vi "Autonomous Independent-old.vi"() -> ()   [LabVIEW 2013]
doc: "This VI is called when autonomous begins, and will automatically be terminated when autonomous ends. You can carry out timed or sensor driven robot movement independently without needing to return to the caller."
uses:
  <vilib>/Rock Robotics/WPI/Solenoid/WPI_SolenoidValue.ctl
  Robot Global Data.vi
  <vilib>/Rock Robotics/WPI/Solenoid/WPI_SolenoidSetEnum.vi
  <vilib>/Rock Robotics/WPI/RobotDrive/WPI_RobotDriveArcadeDrive_Standard(NoSaturation).vi
  <vilib>/Rock Robotics/WPI/RobotDrive/WPI_RobotDriveGetSetRefNum.vi
  <vilib>/Rock Robotics/WPI/Joystick/WPI_JoystickGetSetRefNum.vi
  <vilib>/addons/control/pid/NI_PID_pid.lvlib
  <vilib>/addons/control/pid/pid.llb/PID (DBL).vi
  TargetType.ctl
panel:
  out "Go now or wait?":enum16{"Go Now", "Wait"}(ring)
  out "Stop Time":u32=1000
  in  "stop":bool
  out "Drive Forward Time":u32=1000
  out "Shoot Time":u32=1000
  out "Right? (T)":bool
  out "Position":T1
  in  "Launcher State":enum16{"Shoot", "Out", "Retract"}(ring)
  in  "Shooter Extended Time":u32=500
  out "Shooter Tick":u32
  out "Check Target Time":u32=5000
  out "Left?":bool
  out "Raise Arms Time":u32=1500
  in  "Up Position":dbl format="%.2f"
  out "Close Arms Time":u32=250
  out "Lower Arms Time":u32=1500
  in  "Down Position":dbl format="%.2f"
  out "Open Arms Time":u32=250
  in  "Auton State":T2(ring)
  out "Tick at start of Auton":u32
  out "Current Movement, for debugging":T3 {"Y Joystick Value" scale=1.0..-1.0; "X Joystick Value" scale=-1.0..1.0}
  in  "Array of robot movements":T4(array[cluster]) {"Y Joystick Value" scale=1.0..-1.0; "X Joystick Value" scale=-1.0..1.0}
  # "Be sure to right-click and choose Data Operations>>Make Current Value default if you want to save the array values with the VI"
  # "Main State Machine"
  # "Shooter State Machine"
  # "Disabled"
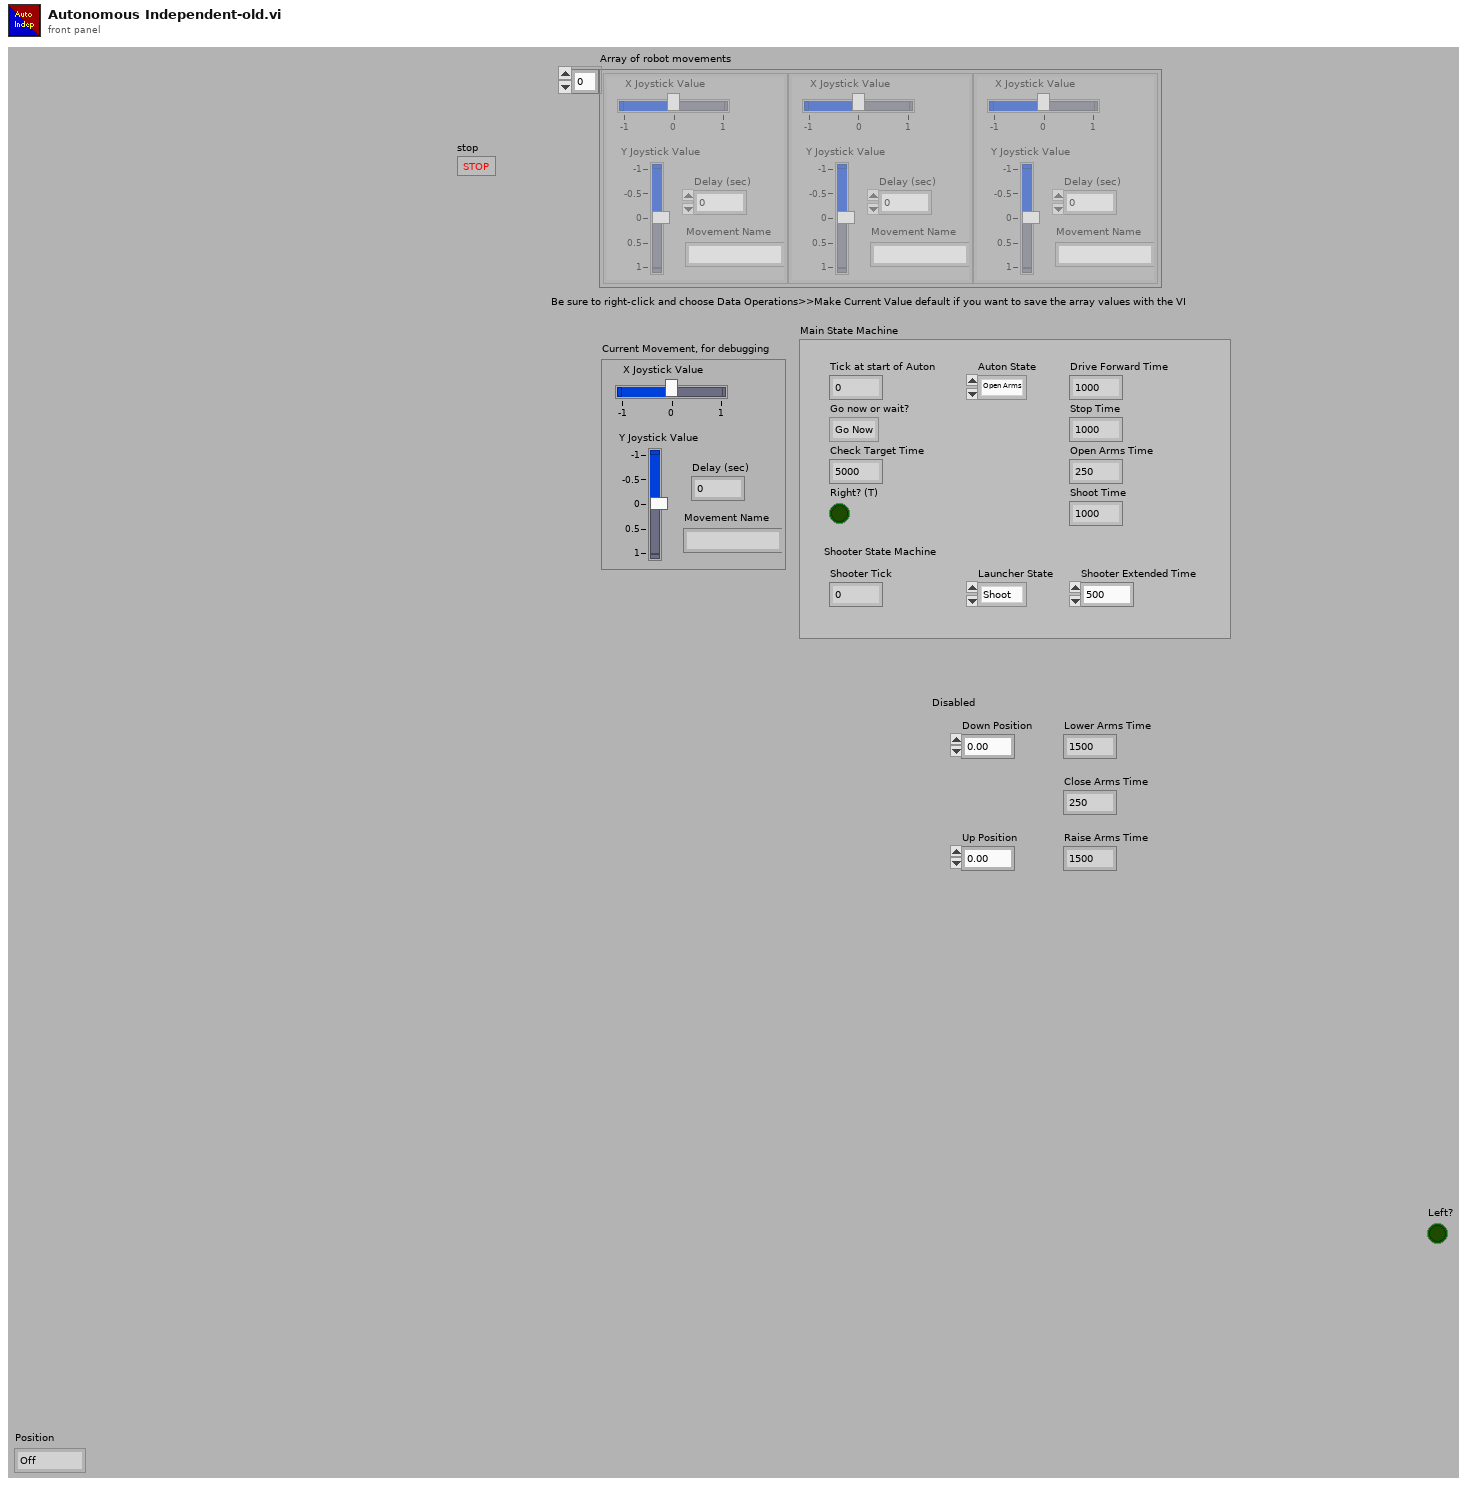
[diagram p1: front panel]
types:
  T1 = typedef "WPI_SolenoidValue.ctl" = enum16{"Off", "On", "Forward", "Reverse"}
  T2 = enum16{"Open Arms", "Lower Arms", "Close Arms", "Raise Arms", "Check Target", "Shoot", "Drive Forward", "Stop"}
  T3 = cluster{"X Joystick Value":dbl, "Y Joystick Value":dbl, "Delay (sec)":dbl, "Movement Name":string}
  T4 = cluster{"X Joystick Value":dbl, "Y Joystick Value":dbl, "Delay (sec)":dbl, "Movement Name":string}[]
  T5 = typedef "WPI_JoystickDevRef.ctl" = cluster{"Device":T6}
  T6 = typedef "WPI_JoystickDeviceEnum.ctl" = enum16{"USB 1", "USB 2", "USB 3", "USB 4", "Kinect 1", "Kinect 2"}
  T7 = cluster{"axis 1 (x)":dbl, "axis 2 (y)":dbl, "axis 3 (throttle)":dbl, "axis 4":dbl, "axis 5":dbl, "axis 6":dbl}
  T8 = typedef "TargetType.ctl" = enum16{"Not Hot", "Hot"}
  T9 = enum16{"Open Arms", "Lower Arms", "Close Arms", "Raise Arms", "Check Target", "Shoot", "Drive Forward"}
  T10 = cluster{"proportional gain (Kc)":dbl, "integral time (Ti, min)":dbl, "derivative time (Td, min)":dbl}
  T11 = typedef "WPI_SolenoidDevRef.ctl" = cluster{"DevStatus":errorcluster, "Solenoid Module":T12, "Forward Solenoid Channel":T13, "Reverse Solenoid Channel":T13}
  T12 = typedef "FPGA_TypedefSolenoidModule.ctl" = enum16{"Solenoid Module 1", "Solenoid Module 2"}
  T13 = typedef "WPI_SolenoidChannel.ctl" = enum8{"Solenoid 1", "Solenoid 2", "Solenoid 3", "Solenoid 4", "Solenoid 5", "Solenoid 6", "Solenoid 7", "Solenoid 8", "Invalid"}
  T14 = enum16{"Target Right", "No Target", "Target Left"}
  T15 = typedef "WPI_RobotDriveDevRef.ctl" = cluster{"DevStatus":errorcluster, "Motors[]":T16[], "Square Inputs":bool, "Max Output":dbl, "Isochronous":bool}
  T16 = typedef "WPI_MotorControlDeviceRef.ctl" = cluster{"DeviceStatus":errorcluster, "Type":enum16{"PWM", "CAN"}, "PWM":cluster{"Digital Module":T17, "PWM Channel":T18, "DeadBand":T19}, "CAN":cluster{"Device Number":u8, "Control Mode":T20, "Semaphore":T21, "Max Vout":dbl}, "Invert":bool, "TransformRef":T22, "InvTransformRef":T22}
  T17 = typedef "FPGA_TypedefDigitalModule.ctl" = enum16{"Digital Module 1", "Digital Module 2"}
  T18 = typedef "FPGA_DIOPWMChannel.ctl" = enum8{"PWM 1", "PWM 2", "PWM 3", "PWM 4", "PWM 5", "PWM 6", "PWM 7", "PWM 8", "PWM 9", "PWM 10", "Invalid"}
  T19 = typedef "WPI_PWMDeadband.ctl" = cluster{"Name":string, "maxPositivePwm":i32, "minPositivePwm":i32, "centerPwm":i32, "maxNegativePwm":i32, "minNegativePwm":i32, "angularRange":u16}
  T20 = typedef "WPI_CANJaguar_ControlMode.ctl" = enum8{"Percent VBus", "Current", "Speed", "Position", "Voltage"}
  T21 = typedef "Semaphore RefNum" = refnum<k1>
  T22 = typedef "WPI_PWMTransform_ConPane.ctl" = refnum<vi>
  T23 = cluster{"Distance (ft)":dbl, "Target Center (-1 to 1)":cluster{"X":dbl, "Y":dbl}, "Left":bool, "State":T8}
  T24 = typedef "WPI_AnalogChannelDevRef.ctl" = cluster{"DevStatus":errorcluster, "Analog Module":T25, "Analog Channel":T26}
  T25 = typedef "FPGA_TypedefAnalogModule.ctl" = enum16{"Analog Module 1", "Analog Module 2"}
  T26 = typedef "FPGA_AIChannel.ctl" = enum8{"AI 1", "AI 2", "AI 3", "AI 4", "AI 5", "AI 6", "AI 7", "AI 8", "Invalid"}
  T27 = typedef "WPI_DigitalInputDevRef.ctl" = cluster{"DevStatus":errorcluster, "DIO Channel":T28, "Digital Module":T17}
  T28 = typedef "FPGA_DIOChannel.ctl" = enum8{"DIO 1", "DIO 2", "DIO 3", "DIO 4", "DIO 5", "DIO 6", "DIO 7", "DIO 8", "DIO 9", "DIO 10", "DIO 11", "DIO 12", "DIO 13", "DIO 14", "Invalid"}
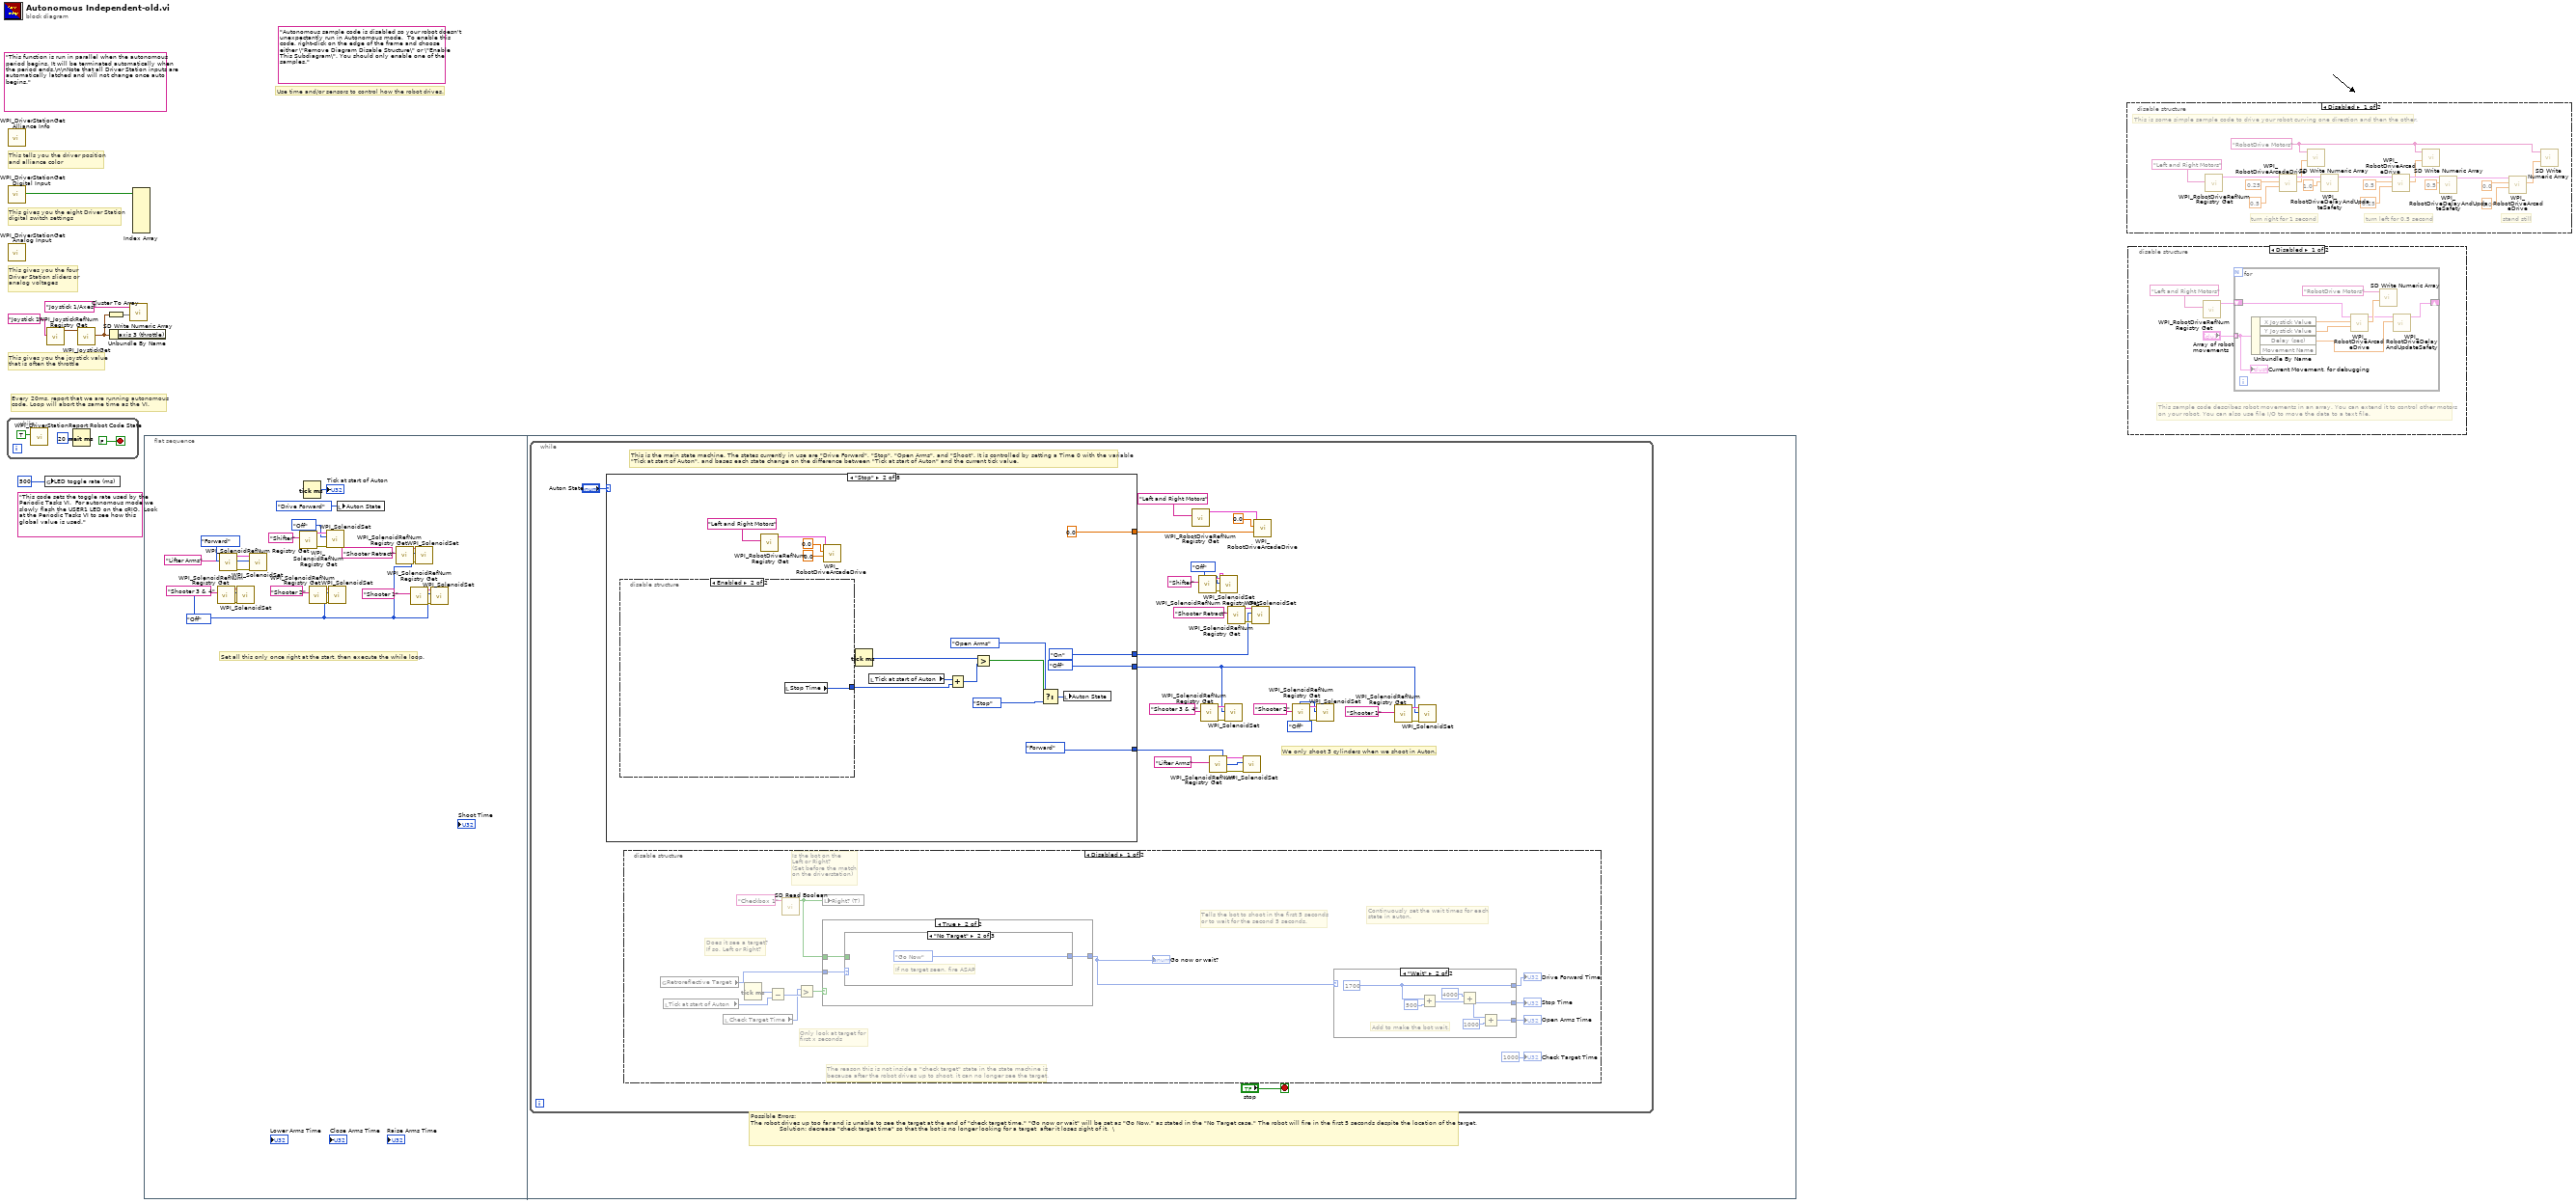
[diagram p0: block diagram]
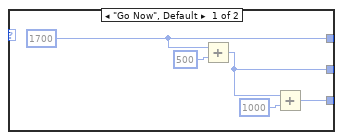
[diagram p2: hidden frame]
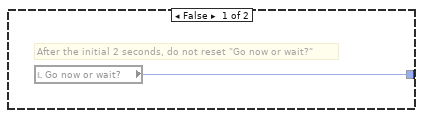
[diagram p3: hidden frame]
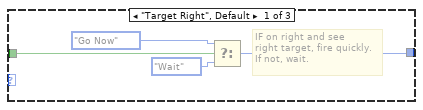
[diagram p4: hidden frame]
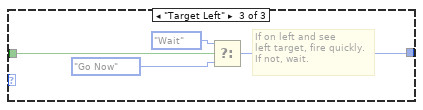
[diagram p5: hidden frame]
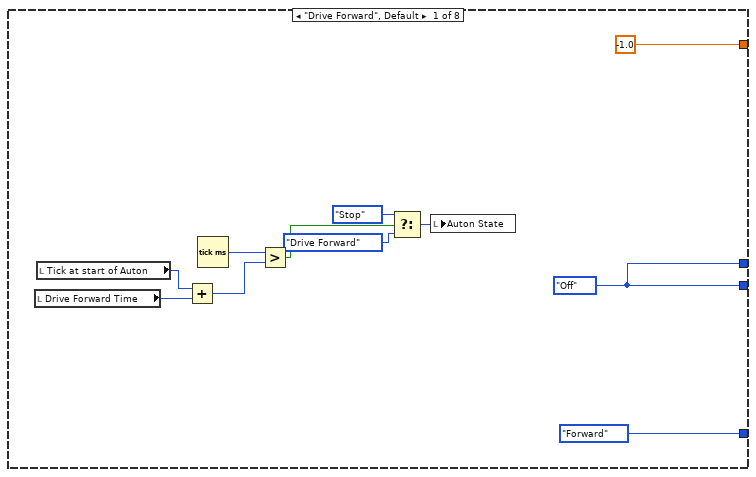
[diagram p7: hidden frame]
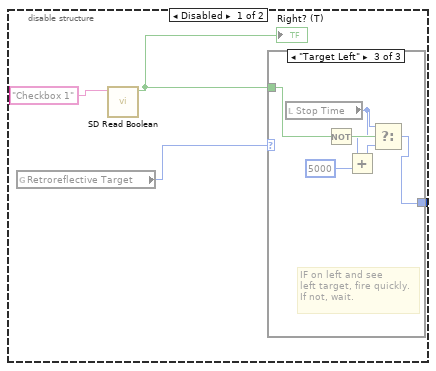
[diagram p8: hidden frame]
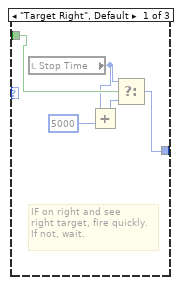
[diagram p9: hidden frame]
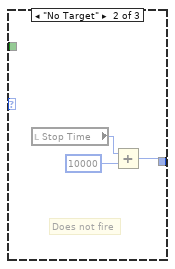
[diagram p10: hidden frame]
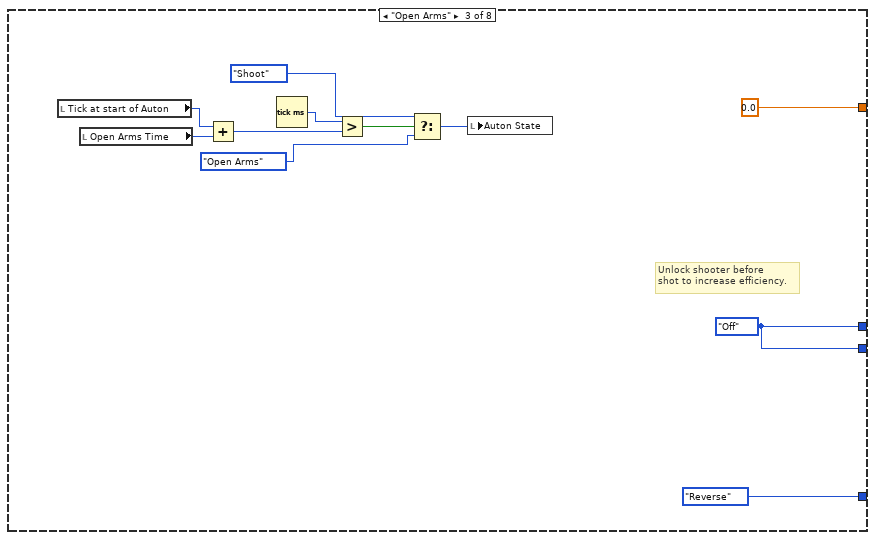
[diagram p11: hidden frame]
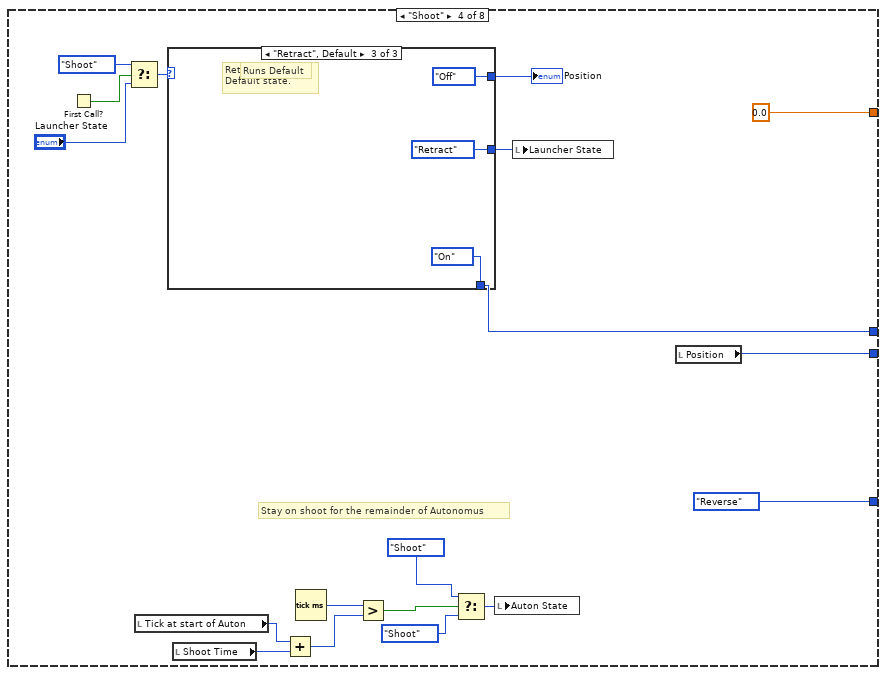
[diagram p12: hidden frame]
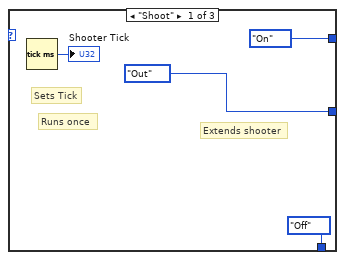
[diagram p13: hidden frame]
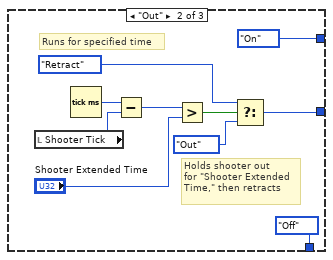
[diagram p14: hidden frame]
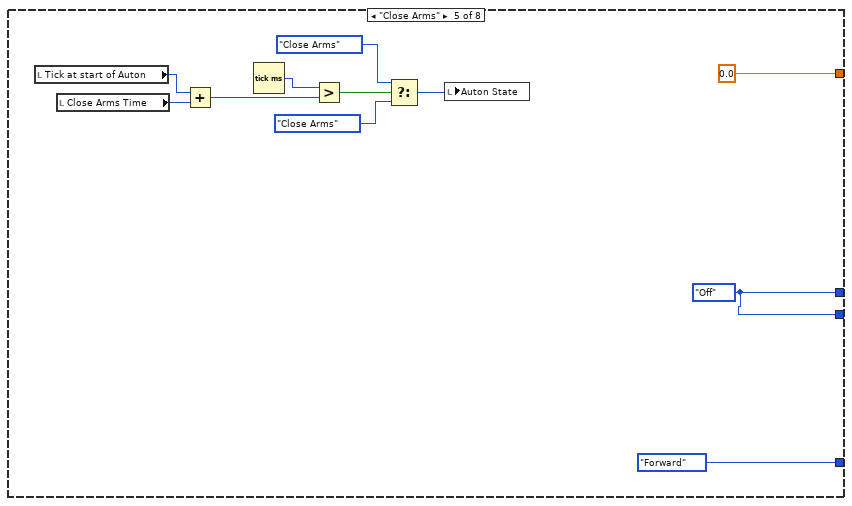
[diagram p15: hidden frame]
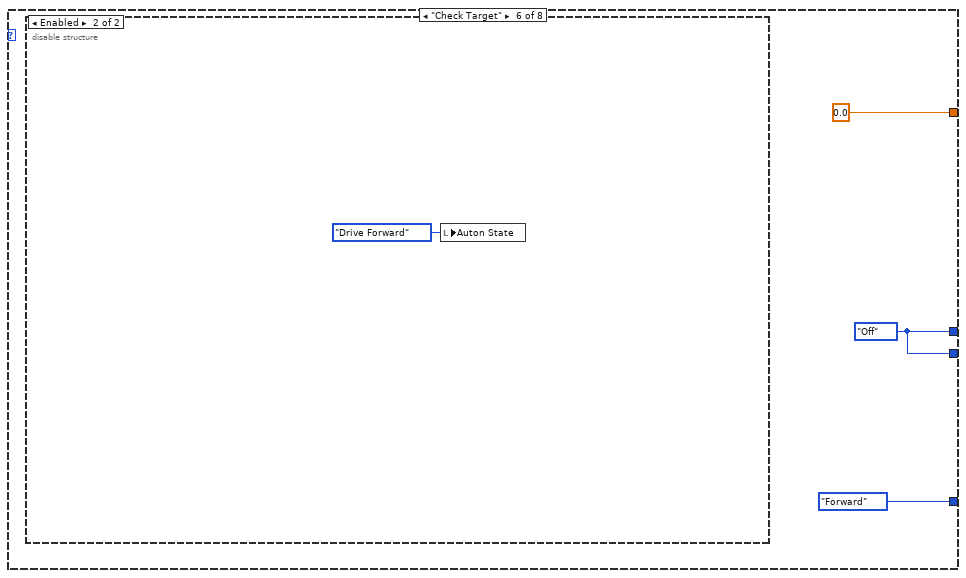
[diagram p16: hidden frame]
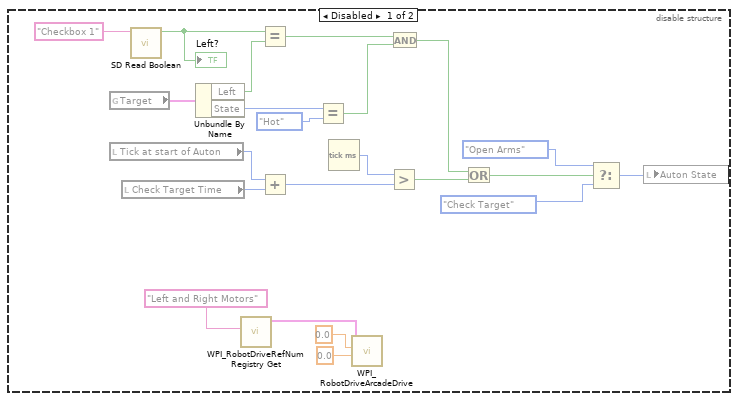
[diagram p17: hidden frame]
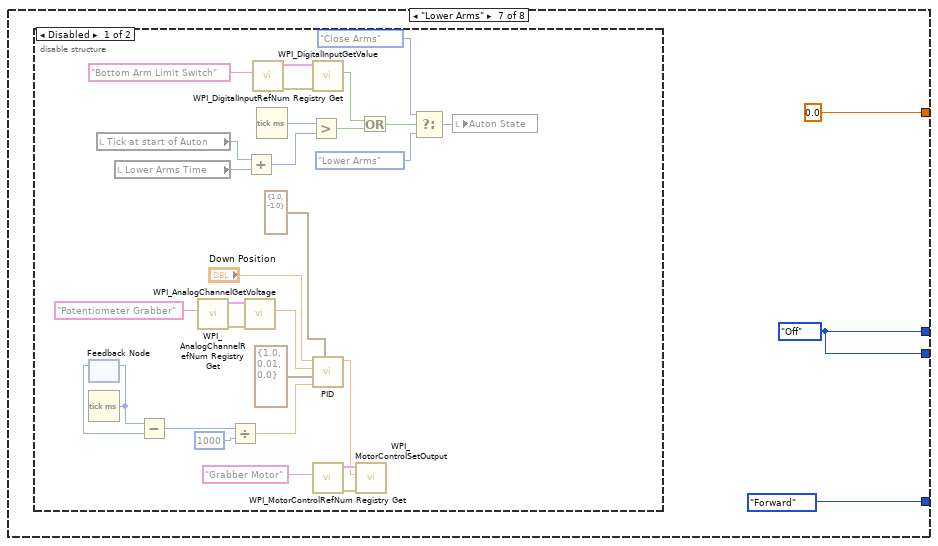
[diagram p18: hidden frame]
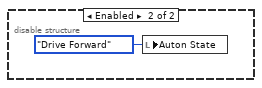
[diagram p19: hidden frame]
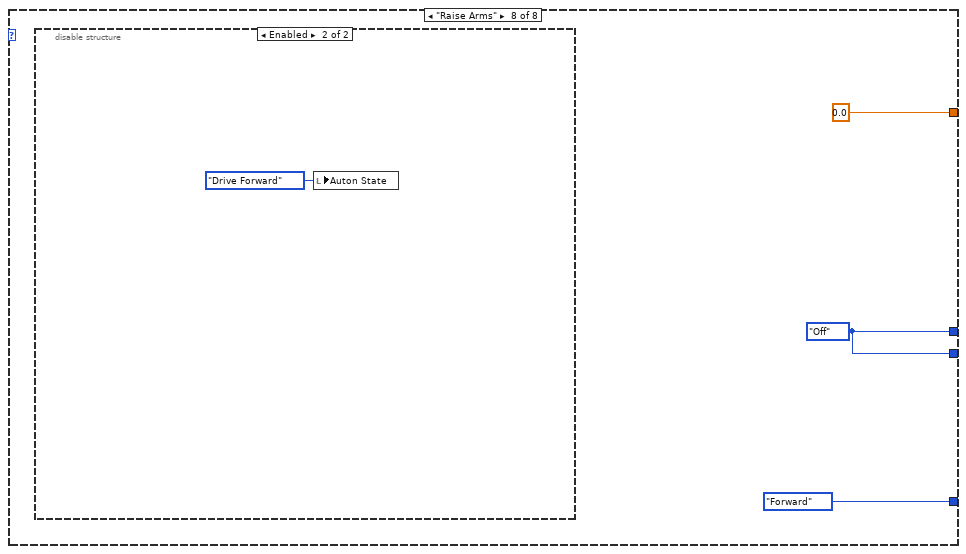
[diagram p20: hidden frame]
diagram:
  (unwired) "This code sets the toggle rate used by the Periodic Tasks VI.  For autonomous mode we slowly flash the USER1 LED on the cRIO.  Look at the Periodic Tasks VI to see how this global value is used."
  (unwired) "Autonomous sample code is disabled so your robot doesn't unexpectantly run in Autonomous mode.  To enable this code, right-click on the edge of the frame and choose either \"Remove Diagram Disable Structure\" or \"Enable This Subdiagram\". You should only enable one of the samples."
  (unwired) "This function is run in parallel when the autonomous period begins. It will be terminated automatically when the period ends.\n\nNote that all Driver Station inputs are automatically latched and will not change once auto begins."
  # "Every 20ms, report that we are running autonomous\ncode. Loop will abort the same time as the VI."
  # "This gives you the joystick value\nthat is often the throttle"
  # "Use time and/or sensors to control how the robot drives."
  # "This tells you the driver position\nand alliance color"
  # "This gives you the eight Driver Station\ndigital switch settings"
  # "This gives you the four\nDriver Station sliders or\nanalog voltages"
  n1 = while {
    stop <- FALSE stop-if-true
    n2 = call <vilib>:"WPI_DriverStationReport Robot Code State.vi"("Autonomous"=TRUE) -> ()  [unwired: 10 in, 1 out]
    n3 = Wait (ms)(milliseconds to wait=u32 20) -> ()  [unwired: 1 out]
  }
  n4 = call <vilib>:"WPI_DriverStationGet Alliance Info.vi"() -> ()  [unwired: 12 out]
  n5 = call <vilib>:"WPI_DriverStationGet Digital Input.vi"() -> ("Driver Station Digital Input (1-8)"=w7:bool[])  [unwired: 11 out]
  n6 = call <vilib>:"WPI_DriverStationGet Analog Input.vi"() -> ()  [unwired: 12 out]
  n7 = global write "Robot Global Data.vi" "LED toggle rate (ms)"(u32 500 ("LED ms toggle rate")) -> ()
  n8 = call <vilib>:"WPI_JoystickRefNum Registry Get.vi"("refnum name"="Joystick 1") -> ("JoystickDevRef"=w5:T5)  [unwired: 1 in, 9 out]
  n9 = call <vilib>:"WPI_JoystickGet.vi"("JoystickDevRef"=w5) -> ("Axes"=w2:T7)  [unwired: 1 in, 5 out]
  n10 = Cluster To Array(cluster=w2) -> (array=w3:dbl[])
  n11 = Unbundle By Name(w2) -> ()  [unwired: 1 out]
  n12 = call <vilib>:"SD Write Numeric Array.vi"("Numeric Array"=w3, "Name"="Joystick 1/Axes") -> ()  [unwired: 8 in, 2 out]
  n13 = Index Array(array=w7) -> ()  [unwired: 8 in, 8 out]
  n14 = flat-sequence {
    frame #0 {
      w19 = WPI_SolenoidValue."Off" ("x")
      # "Set all this only once right at the start, then execute the while loop."
      n15 = call <vilib>:"WPI_SolenoidRefNum Registry Get.vi"("refnum name"="Shooter 3 & 4") -> ("error out"=w26:errorcluster, "SolenoidDevRef"=w30:T11)  [unwired: 9 in]
      n16 = call <vilib>:"WPI_SolenoidRefNum Registry Get.vi"("refnum name"="Lifter Arms") -> ("error out"=w13:errorcluster, "SolenoidDevRef"=w14:T11)  [unwired: 9 in]
      n17 = call-poly <vilib>:"WPI_SolenoidSet.vi"("error in (no error)"=w26, "Value"=w19, "SolenoidDevRef"=w30) -> ()  [unwired: 7 in, 2 out]
      n18 = call-poly <vilib>:"WPI_SolenoidSet.vi"("error in (no error)"=w13, "Value"=WPI_SolenoidValue."Forward", "SolenoidDevRef"=w14) -> ()  [unwired: 7 in, 2 out]
      n19 = call <vilib>:"WPI_SolenoidRefNum Registry Get.vi"("refnum name"="Shifter") -> ("error out"=w17:errorcluster, "SolenoidDevRef"=w16:T11)  [unwired: 9 in]
      n20 = Tick Count (ms)() -> (millisecond timer value=→"Tick at start of Auton":u32)
      n21 = call <vilib>:"WPI_SolenoidRefNum Registry Get.vi"("refnum name"="Shooter 2") -> ("error out"=w23:errorcluster, "SolenoidDevRef"=w31:T11)  [unwired: 9 in]
      n22 = call-poly <vilib>:"WPI_SolenoidSet.vi"("error in (no error)"=w17, "Value"=WPI_SolenoidValue."Off", "SolenoidDevRef"=w16) -> ()  [unwired: 7 in, 2 out]
      n23 = call-poly <vilib>:"WPI_SolenoidSet.vi"("error in (no error)"=w23, "Value"=w19, "SolenoidDevRef"=w31) -> ()  [unwired: 7 in, 2 out]
      n24 = local write "Auton State"(T2."Drive Forward" ("Auton State")) -> ()
      n25 = call <vilib>:"WPI_SolenoidRefNum Registry Get.vi"("refnum name"="Shooter Retract") -> ("error out"=w21:errorcluster, "SolenoidDevRef"=w20:T11)  [unwired: 9 in]
      n26 = call <vilib>:"WPI_SolenoidRefNum Registry Get.vi"("refnum name"="Shooter 1") -> ("error out"=w28:errorcluster, "SolenoidDevRef"=w29:T11)  [unwired: 9 in]
      n27 = call-poly <vilib>:"WPI_SolenoidSet.vi"("error in (no error)"=w21, "Value"=w19, "SolenoidDevRef"=w20) -> ()  [unwired: 7 in, 2 out]
      n28 = call-poly <vilib>:"WPI_SolenoidSet.vi"("error in (no error)"=w28, "Value"=w19, "SolenoidDevRef"=w29) -> ()  [unwired: 7 in, 2 out]
    }
    frame #1 {
      # "Possible Errors:\nThe robot drives up too far and is unable to see the target at the end of \"check target time.\" \"Go now or wait\" will be set as \"Go Now,\" as stated in the \"No Target case.\" The robot will fire in the first 5 seconds despite the location of the target.\n               Solution: decrease \"check target time\" so that the bot is no longer looking for a target  after it loses sight of it.  \\"
      n29 = while {
        stop <- "stop" stop-if-true
        # "We only shoot 3 cylinders when we shoot in Auton."
        # "This is the main state machine. The states currently in use are \"Drive Forward\", \"Stop\", \"Open Arms\", and \"Shoot\". It is controlled by setting a Time 0 with the variable\n\"Tick at start of Auton\", and bases each state change on the difference between \"Tick at start of Auton\" and the current tick value."
        n30 = case shown="\"Stop\"" "Auton State" {
          tunnel: [w103 WPI_SolenoidValue."Off" ("x") w149 w161 w197 w204 w232 w265] -> w48
          tunnel: [w103 WPI_SolenoidValue."On" ("x") w149 w158 w197 w204 w232 w265] -> w47
          tunnel: [-1.0 ("Y axis value") 0.0 ("Y axis value") 0.0 ("Y axis value") 0.0 ("Y axis value") 0.0 ("Y axis value") 0.0 ("Y axis value") 0.0 ("Y axis value") 0.0 ("Y axis value")] -> w43
          tunnel: [WPI_SolenoidValue."Forward" ("Value") WPI_SolenoidValue."Forward" ("Value") WPI_SolenoidValue."Reverse" ("Value") WPI_SolenoidValue."Reverse" ("Value") WPI_SolenoidValue."Forward" ("Value") WPI_SolenoidValue."Forward" ("Value") WPI_SolenoidValue."Forward" ("Value") WPI_SolenoidValue."Forward" ("Value")] -> w35
          frame "Drive Forward", Default {
            w103 = WPI_SolenoidValue."Off" ("Value")
            n31 = local read "Drive Forward Time"() -> (w111:u32)
            n32 = local read "Tick at start of Auton"() -> (w109:u32)
            n33 = Add(x=w109, y=w111) -> (x+y=w110:u32)
            n34 = Tick Count (ms)() -> (millisecond timer value=w108:u32)
            n35 = Greater?(x=w108, y=w110) -> (0:w106:bool)
            n36 = Select(t=T2."Stop" ("Auton State"), s=w106, f=T2."Drive Forward" ("Auton State")) -> (s? t:f=w107:T2)
            n37 = local write "Auton State"(w107) -> ()
          }
          frame "Stop" {
            n38 = disable-structure shown="Enabled" {
              disable-tunnel: [w128 w146] -> w112
              frame Disabled {
                n39 = global read "Robot Global Data.vi" "Retroreflective Target"() -> (w130:T14)
                n40 = call <vilib>:"SD Read Boolean.vi"("Name"="Checkbox 1" ("refnum name")) -> ("Boolean"=w129:bool)  [unwired: 8 in, 2 out]
                "Right? (T)" <- w129
                n41 = case shown="\"Target Left\"" w130 {
                  tunnel: w129 -> [w133 _ w145]
                  tunnel: [w134 w139 w140] -> w128
                  frame "Target Right", Default {
                    # "IF on right and see\nright target, fire quickly.\nIf not, wait."
                    n42 = local read "Stop Time"() -> (w132:u32)
                    n43 = Add(x=w132, y=u32 5000) -> (x+y=w136:u32)
                    n44 = Select(t=w132, s=w133, f=w136) -> (s? t:f=w134:u32)
                  }
                  frame "No Target" {
                    # "Does not fire"
                    n45 = local read "Stop Time"() -> (w138:u32)
                    n46 = Add(x=w138, y=u32 10000) -> (x+y=w139:u32)
                  }
                  frame "Target Left" {
                    # "IF on left and see\nleft target, fire quickly.\nIf not, wait."
                    n47 = local read "Stop Time"() -> (w143:u32)
                    n48 = Not(x=w145) -> (.not. x?=w144:bool)
                    n49 = Add(x=w143, y=u32 5000) -> (x+y=w142:u32)
                    n50 = Select(t=w143, s=w144, f=w142) -> (s? t:f=w140:u32)
                  }
                }
              }
              frame Enabled {
                n51 = local read "Stop Time"() -> (w146:u32)
              }
            }
            n52 = call <vilib>:"WPI_RobotDriveRefNum Registry Get.vi"("refnum name"="Left and Right Motors") -> ("RobotDriveDevRef"=w124:T15)  [unwired: 1 in, 9 out]
            n53 = call-poly <vilib>:"WPI_RobotDriveArcadeDrive.vi"("Y axis value"=0.0, "X axis value"=0.0, "RobotDriveDevRef"=w124) -> ()  [unwired: 6 in, 3 out]
            n54 = Tick Count (ms)() -> (millisecond timer value=w118:u32)
            n55 = local read "Tick at start of Auton"() -> (w119:u32)
            n56 = Add(x=w119, y=w112) -> (x+y=w120:u32)
            n57 = Greater?(x=w118, y=w120) -> (0:w116:bool)
            n58 = Select(t=T2."Open Arms" ("Auton State"), s=w116, f=T2."Stop" ("Auton State")) -> (s? t:f=w117:T2)
            n59 = local write "Auton State"(w117) -> ()
          }
          frame "Open Arms" {
            w149 = WPI_SolenoidValue."Off" ("Value")
            # "Unlock shooter before\nshot to increase efficiency."
            n60 = local read "Tick at start of Auton"() -> (w156:u32)
            n61 = local read "Open Arms Time"() -> (w153:u32)
            n62 = Add(x=w156, y=w153) -> (x+y=w155:u32)
            n63 = Tick Count (ms)() -> (millisecond timer value=w157:u32)
            n64 = Greater?(x=w157, y=w155) -> (0:w154:bool)
            n65 = Select(t=T2."Shoot" ("Auton State"), s=w154, f=T2."Open Arms" ("Auton State")) -> (s? t:f=w150:T2)
            n66 = local write "Auton State"(w150) -> ()
          }
          frame "Shoot" {
            # "Stay on shoot for the remainder of Autonomus"
            n67 = First Call?() -> (First Call?: T/F=w170:bool)
            n68 = Select(t=enum16{"Shoot", "Out", "Retract"}."Shoot", s=w170, f="Launcher State") -> (s? t:f=w174:enum16{"Shoot", "Out", "Retract"})
            n69 = local read "Tick at start of Auton"() -> (w167:u32)
            n70 = case shown="\"Retract\", Default" w174 {
              tunnel: [WPI_SolenoidValue."On" ("Value") WPI_SolenoidValue."On" ("Value") WPI_SolenoidValue."Off" ("Value")] -> w171
              tunnel: [enum16{"Shoot", "Out", "Retract"}."Out" ("Launcher State") w182 enum16{"Shoot", "Out", "Retract"}."Retract" ("Launcher State")] -> w172
              tunnel: [WPI_SolenoidValue."Off" ("t") WPI_SolenoidValue."Off" ("t") WPI_SolenoidValue."On" ("t")] -> w158
              frame "Shoot" {
                # "Runs once"
                # "Sets Tick"
                # "Extends shooter"
                n71 = Tick Count (ms)() -> (millisecond timer value=→"Shooter Tick":u32)
              }
              frame "Out" {
                # "Runs for specified time"
                # "Holds shooter out\nfor \"Shooter Extended\nTime,\" then retracts"
                n72 = local read "Shooter Tick"() -> (w188:u32)
                n73 = Tick Count (ms)() -> (millisecond timer value=w189:u32)
                n74 = Subtract(x=w189, y=w188) -> (x-y=w187:u32)
                n75 = Greater?(x=w187, y="Shooter Extended Time") -> (0:w186:bool)
                n76 = Select(t=enum16{"Shoot", "Out", "Retract"}."Retract" ("Launcher State"), s=w186, f=enum16{"Shoot", "Out", "Retract"}."Out" ("Launcher State")) -> (s? t:f=w182:enum16{"Shoot", "Out", "Retract"})
              }
              frame "Retract", Default {
                # "Runs Default"
                # "Retracts Shooter, \nDefault state."
              }
            }
            "Position" <- w171
            n77 = local read "Shoot Time"() -> (w169:u32)
            n78 = Add(x=w167, y=w169) -> (x+y=w168:u32)
            n79 = Tick Count (ms)() -> (millisecond timer value=w166:u32)
            n80 = Greater?(x=w166, y=w168) -> (0:w164:bool)
            n81 = Select(t=T2."Shoot" ("Auton State"), s=w164, f=T2."Shoot" ("Auton State")) -> (s? t:f=w165:T2)
            n82 = local write "Auton State"(w165) -> ()
            n83 = local write "Launcher State"(w172) -> ()
            n84 = local read "Position"() -> (w161:T1)
          }
          frame "Close Arms" {
            w197 = WPI_SolenoidValue."Off" ("x")
            n85 = local read "Tick at start of Auton"() -> (w200:u32)
            n86 = local read "Close Arms Time"() -> (w203:u32)
            n87 = Add(x=w200, y=w203) -> (x+y=w201:u32)
            n88 = Tick Count (ms)() -> (millisecond timer value=w199:u32)
            n89 = Greater?(x=w199, y=w201) -> (0:w202:bool)
            n90 = Select(t=T2."Close Arms" ("Auton State"), s=w202, f=T2."Close Arms" ("Auton State")) -> (s? t:f=w198:T2)
            n91 = local write "Auton State"(w198) -> ()
          }
          frame "Check Target" {
            w204 = WPI_SolenoidValue."Off" ("x")
            n92 = disable-structure shown="Enabled" {
              frame Disabled {
                n93 = global read "Robot Global Data.vi" "Target"() -> (w228:T23)
                n94 = local read "Tick at start of Auton"() -> (w216:u32)
                n95 = local read "Check Target Time"() -> (w218:u32)
                n96 = call <vilib>:"SD Read Boolean.vi"("Name"="Checkbox 1" ("refnum name")) -> ("Boolean"=w223:bool)  [unwired: 8 in, 2 out]
                "Left?" <- w223
                n97 = Unbundle By Name(w228) -> ("Left"=w224:bool, "State"=w227:T8)
                n98 = call <vilib>:"WPI_RobotDriveRefNum Registry Get.vi"("refnum name"="Left and Right Motors") -> ("RobotDriveDevRef"=w209:T15)  [unwired: 1 in, 9 out]
                n99 = Equal?(x=w223, y=w224) -> (x = y?=w221:bool)
                n100 = Add(x=w216, y=w218) -> (x+y=w217:u32)
                n101 = Equal?(x=w227, y=TargetType."Hot") -> (x = y?=w222:bool)
                n102 = Tick Count (ms)() -> (millisecond timer value=w215:u32)
                n103 = call-poly <vilib>:"WPI_RobotDriveArcadeDrive.vi"("Y axis value"=0.0, "X axis value"=0.0, "RobotDriveDevRef"=w209) -> ()  [unwired: 6 in, 3 out]
                n104 = Greater?(x=w215, y=w217) -> (0:w220:bool)
                n105 = And(x=w221, y=w222) -> (x .and. y?=w213:bool)
                n106 = Or(x=w213, y=w220) -> (x .or. y?=w219:bool)
                n107 = Select(t=T2."Open Arms" ("Auton State"), s=w219, f=T2."Check Target" ("Auton State")) -> (s? t:f=w214:T2)
                n108 = local write "Auton State"(w214) -> ()
              }
              frame Enabled {
                n109 = local write "Auton State"(T2."Drive Forward" ("Auton State")) -> ()
              }
            }
          }
          frame "Lower Arms" {
            w232 = WPI_SolenoidValue."Off" ("x")
            n110 = disable-structure shown="Disabled" {
              frame Disabled {
                n111 = feedback #1() -> (w256:u32)  [unwired: 1 in]
                n112 = Tick Count (ms)() -> (millisecond timer value=w257:u32)
                n113 = feedback-in #1(w257) -> ()
                n114 = local read "Tick at start of Auton"() -> (w238:u32)
                n115 = local read "Lower Arms Time"() -> (w236:u32)
                n116 = Subtract(x=w257, y=w256) -> (x-y=w255:u32)
                n117 = call <vilib>:"WPI_AnalogChannelRefNum Registry Get.vi"("refnum name"="Potentiometer Grabber") -> ("error out"=w259:errorcluster, "AIDeviceRef"=w260:T24)  [unwired: 9 in]
                n118 = Divide(x=w255, y=u32 1000) -> (x/y=w253:dbl)
                n119 = call <vilib>:"WPI_AnalogChannelGetVoltage.vi"("error in (no error)"=w259, "AIDeviceRef"=w260) -> ("Voltage"=w247:dbl)  [unwired: 7 in, 2 out]
                n120 = Add(x=w238, y=w236) -> (x+y=w237:u32)
                n121 = call <vilib>:"WPI_DigitalInputRefNum Registry Get.vi"("refnum name"="Bottom Arm Limit Switch") -> ("error out"=w242:errorcluster, "DigitalInputDevRef"=w241:T27)  [unwired: 9 in]
                n122 = Tick Count (ms)() -> (millisecond timer value=w239:u32)
                n123 = Greater?(x=w239, y=w237) -> (0:w233:bool)
                n124 = call <vilib>:"WPI_DigitalInputGetValue.vi"("error in (no error)"=w242, "DigitalInputDevRef"=w241) -> ("Value"=w234:bool)  [unwired: 7 in, 2 out]
                n125 = call-poly <vilib>:"PID.vi"("output range"=cluster{"output high":dbl, "output low":dbl} {"output high"=1.0, "output low"=-1.0}, "dt (s)"=w253, "PID gains"=T10 {"proportional gain (Kc)"=1.0, "integral time (Ti, min)"=0.01, "derivative time (Td, min)"=0.0}, "process variable"=w247, "setpoint"="Down Position") -> ("output"=w250:dbl)  [unwired: 5 in, 1 out]
                n126 = call <vilib>:"WPI_MotorControlRefNum Registry Get.vi"("refnum name"="Grabber Motor") -> ("error out"=w252:errorcluster, "MotorControlDevRef"=w251:T16)  [unwired: 9 in]
                n127 = call <vilib>:"WPI_MotorControlSetOutput.vi"("error in (no error)"=w252, "Output"=w250, "MotorControlDevRef"=w251) -> ()  [unwired: 6 in, 3 out]
                n128 = Or(x=w234, y=w233) -> (x .or. y?=w235:bool)
                n129 = Select(t=T9."Close Arms", s=w235, f=T9."Lower Arms") -> (s? t:f=w245:T9)
                n130 = local write "Auton State"(w245) -> ()
              }
              frame Enabled {
                n131 = local write "Auton State"(T2."Drive Forward" ("Auton State")) -> ()
              }
            }
          }
          frame "Raise Arms" {
            w265 = WPI_SolenoidValue."Off" ("x")
            n132 = disable-structure shown="Enabled" {
              frame Disabled {
                n133 = feedback #2() -> (w271:u32)  [unwired: 1 in]
                n134 = Tick Count (ms)() -> (millisecond timer value=w270:u32)
                n135 = feedback-in #2(w270) -> ()
                n136 = local read "Tick at start of Auton"() -> (w289:u32)
                n137 = local read "Raise Arms Time"() -> (w291:u32)
                n138 = Subtract(x=w270, y=w271) -> (x-y=w272:u32)
                n139 = call <vilib>:"WPI_AnalogChannelRefNum Registry Get.vi"("refnum name"="Potentiometer Grabber") -> ("error out"=w268:errorcluster, "AIDeviceRef"=w267:T24)  [unwired: 9 in]
                n140 = Divide(x=w272, y=u32 1000) -> (x/y=w274:dbl)
                n141 = call <vilib>:"WPI_AnalogChannelGetVoltage.vi"("error in (no error)"=w268, "AIDeviceRef"=w267) -> ("Voltage"=w280:dbl)  [unwired: 7 in, 2 out]
                n142 = Add(x=w289, y=w291) -> (x+y=w290:u32)
                n143 = call <vilib>:"WPI_DigitalInputRefNum Registry Get.vi"("refnum name"="Top Arm Limit Switch") -> ("error out"=w285:errorcluster, "DigitalInputDevRef"=w286:T27)  [unwired: 9 in]
                n144 = Tick Count (ms)() -> (millisecond timer value=w288:u32)
                n145 = Greater?(x=w288, y=w290) -> (0:w294:bool)
                n146 = call <vilib>:"WPI_DigitalInputGetValue.vi"("error in (no error)"=w285, "DigitalInputDevRef"=w286) -> ("Value"=w293:bool)  [unwired: 7 in, 2 out]
                n147 = call-poly <vilib>:"PID.vi"("output range"=cluster{"output high":dbl, "output low":dbl} {"output high"=1.0, "output low"=-1.0}, "dt (s)"=w274, "PID gains"=T10 {"proportional gain (Kc)"=1.0, "integral time (Ti, min)"=0.01, "derivative time (Td, min)"=0.0}, "process variable"=w280, "setpoint"="Up Position") -> ("output"=w277:dbl)  [unwired: 5 in, 1 out]
                n148 = call <vilib>:"WPI_MotorControlRefNum Registry Get.vi"("refnum name"="Grabber Motor") -> ("error out"=w275:errorcluster, "MotorControlDevRef"=w276:T16)  [unwired: 9 in]
                n149 = call <vilib>:"WPI_MotorControlSetOutput.vi"("error in (no error)"=w275, "Output"=w277, "MotorControlDevRef"=w276) -> ()  [unwired: 6 in, 3 out]
                n150 = Or(x=w293, y=w294) -> (x .or. y?=w292:bool)
                n151 = Select(t=T9."Check Target", s=w292, f=T9."Raise Arms") -> (s? t:f=w282:T9)
                n152 = local write "Auton State"(w282) -> ()
              }
              frame Enabled {
                n153 = local write "Auton State"(T2."Drive Forward" ("Auton State")) -> ()
              }
            }
          }
        }
        n154 = disable-structure shown="Disabled" {
          frame Disabled {
            # "The reason this is not inside a \"check target\" state in the state machine is \nbecause after the robot drives up to shoot, it can no longer see the target."
            # "Continuously set the wait times for each\nstate in auton."
            # "Tells the bot to shoot in the first 5 seconds\nor to wait for the second 5 seconds."
            # "Is the bot on the\nLeft or Right?\n(Set before the match\non the driverstation)"
            # "Does it see a target?\nIf so, Left or Right?"
            # "Only look at target for \nfirst x seconds"
            n155 = global read "Robot Global Data.vi" "Retroreflective Target"() -> (w73:T14)
            n156 = local read "Tick at start of Auton"() -> (w71:u32)
            n157 = local read "Check Target Time"() -> (w64:u32)
            n158 = Tick Count (ms)() -> (millisecond timer value=w72:u32)
            n159 = Subtract(x=w72, y=w71) -> (x-y=w70:u32)
            n160 = call <vilib>:"SD Read Boolean.vi"("Name"="Checkbox 1" ("refnum name")) -> ("Boolean"=w74:bool)  [unwired: 8 in, 2 out]
            n161 = Greater?(x=w64, y=w70) -> (0:w69:bool)
            n162 = local write "Right? (T)"(w74) -> ()
            n163 = case shown="True" w69 {
              tunnel: w74 -> [_ w91]
              tunnel: w73 -> [_ w90]
              tunnel: [w88 w89] -> w65
              frame False {
                # "After the initial 2 seconds, do not reset \"Go now or wait?\""
                n164 = local read "Go now or wait?"() -> (w88:enum16{"Go Now", "Wait"})
              }
              frame True {
                n165 = case shown="\"No Target\"" w90 {
                  tunnel: w91 -> [w94 _ w99]
                  tunnel: [w95 enum16{"Go Now", "Wait"}."Go Now" w100] -> w89
                  frame "Target Right", Default {
                    # "IF on right and see\nright target, fire quickly.\nIf not, wait."
                    n166 = Select(t=enum16{"Go Now", "Wait"}."Go Now", s=w94, f=enum16{"Go Now", "Wait"}."Wait") -> (s? t:f=w95:enum16{"Go Now", "Wait"})
                  }
                  frame "No Target" {
                    # "If no target seen, fire ASAP"
                  }
                  frame "Target Left" {
                    # "If on left and see\nleft target, fire quickly.\nIf not, wait."
                    n167 = Select(t=enum16{"Go Now", "Wait"}."Wait", s=w99, f=enum16{"Go Now", "Wait"}."Go Now") -> (s? t:f=w100:enum16{"Go Now", "Wait"})
                  }
                }
              }
            }
            "Go now or wait?" <- w65
            n168 = case shown="\"Wait\"" w65 {
              tunnel: [w78 w82] -> w68
              tunnel: [w77 w81] -> w67
              tunnel: [w76 w84] -> w66
              frame "Go Now", Default {
                w76 = u32 1700 ("Drive Forward Time")
                n169 = Add(x=w76, y=u32 500 ("Drive Forward Time")) -> (x+y=w77:u32)
                n170 = Add(x=w77, y=u32 1000 ("Open Arms Time")) -> (x+y=w78:u32)
              }
              frame "Wait" {
                w84 = u32 1700 ("Drive Forward Time")
                # "Add to make the bot wait."
                n171 = Add(x=w84, y=u32 500 ("Drive Forward Time")) -> (x+y=w83:u32)
                n172 = Add(x=u32 4000, y=w83) -> (x+y=w81:u32)
                n173 = Add(x=w81, y=u32 1000 ("Open Arms Time")) -> (x+y=w82:u32)
              }
            }
            "Open Arms Time" <- w68
            "Drive Forward Time" <- w66
            "Stop Time" <- w67
            "Check Target Time" <- u32 1000 ("Check Target Time")
          }
          frame Enabled {
          }
        }
        n174 = call <vilib>:"WPI_RobotDriveRefNum Registry Get.vi"("refnum name"="Left and Right Motors") -> ("RobotDriveDevRef"=w46:T15)  [unwired: 1 in, 9 out]
        n175 = call <vilib>:"WPI_SolenoidRefNum Registry Get.vi"("refnum name"="Shifter") -> ("error out"=w41:errorcluster, "SolenoidDevRef"=w40:T11)  [unwired: 9 in]
        n176 = call <vilib>:"WPI_SolenoidRefNum Registry Get.vi"("refnum name"="Shooter 3 & 4") -> ("error out"=w55:errorcluster, "SolenoidDevRef"=w59:T11)  [unwired: 9 in]
        n177 = call <vilib>:"WPI_SolenoidRefNum Registry Get.vi"("refnum name"="Lifter Arms") -> ("error out"=w37:errorcluster, "SolenoidDevRef"=w36:T11)  [unwired: 9 in]
        n178 = call-poly <vilib>:"WPI_SolenoidSet.vi"("error in (no error)"=w41, "Value"=WPI_SolenoidValue."Off", "SolenoidDevRef"=w40) -> ()  [unwired: 7 in, 2 out]
        n179 = call-poly <vilib>:"WPI_SolenoidSet.vi"("error in (no error)"=w55, "Value"=w48, "SolenoidDevRef"=w59) -> ()  [unwired: 7 in, 2 out]
        n180 = call <vilib>:"WPI_SolenoidRefNum Registry Get.vi"("refnum name"="Shooter Retract") -> ("error out"=w50:errorcluster, "SolenoidDevRef"=w49:T11)  [unwired: 9 in]
        n181 = call-poly <vilib>:"WPI_SolenoidSet.vi"("error in (no error)"=w37, "Value"=w35, "SolenoidDevRef"=w36) -> ()  [unwired: 7 in, 2 out]
        n182 = call-poly <vilib>:"WPI_SolenoidSet.vi"("error in (no error)"=w50, "Value"=w47, "SolenoidDevRef"=w49) -> ()  [unwired: 7 in, 2 out]
        n183 = call-poly <vilib>:"WPI_RobotDriveArcadeDrive.vi"("Y axis value"=w43, "X axis value"=0.0, "RobotDriveDevRef"=w46) -> ()  [unwired: 6 in, 3 out]
        n184 = call <vilib>:"WPI_SolenoidRefNum Registry Get.vi"("refnum name"="Shooter 2") -> ("error out"=w52:errorcluster, "SolenoidDevRef"=w60:T11)  [unwired: 9 in]
        n185 = call-poly <vilib>:"WPI_SolenoidSet.vi"("error in (no error)"=w52, "Value"=WPI_SolenoidValue."Off", "SolenoidDevRef"=w60) -> ()  [unwired: 7 in, 2 out]
        n186 = call <vilib>:"WPI_SolenoidRefNum Registry Get.vi"("refnum name"="Shooter 1") -> ("error out"=w57:errorcluster, "SolenoidDevRef"=w58:T11)  [unwired: 9 in]
        n187 = call-poly <vilib>:"WPI_SolenoidSet.vi"("error in (no error)"=w57, "Value"=w48, "SolenoidDevRef"=w58) -> ()  [unwired: 7 in, 2 out]
      }
    }
  }
  n188 = disable-structure shown="Disabled" {
    frame Disabled {
      w296 = "RobotDrive Motors" ("Name")
      # "This is some simple sample code to drive your robot curving one direction and then the other."
      # "stand still"
      # "turn left for 0.5 second"
      # "turn right for 1 second"
      n189 = call <vilib>:"WPI_RobotDriveRefNum Registry Get.vi"("refnum name"="Left and Right Motors") -> ("RobotDriveDevRef"=w300:T15)  [unwired: 1 in, 9 out]
      n190 = call-poly <vilib>:"WPI_RobotDriveArcadeDrive.vi"("Y axis value"=0.5 ("X axis value"), "X axis value"=0.25, "RobotDriveDevRef"=w300) -> ("Motor Values"=w299:dbl[], "RobotDriveDevRef"=w307:T15)  [unwired: 1 in, 6 out]
      n191 = call <vilib>:"SD Write Numeric Array.vi"("Numeric Array"=w299, "Name"=w296) -> ()  [unwired: 8 in, 2 out]
      n192 = call <vilib>:"WPI_RobotDriveDelayAndUpdateSafety.vi"("Delay (s)"=1.0, "RobotDriveDevRef"=w307) -> ("RobotDriveDevRef 2"=w306:T15)  [unwired: 8 in, 1 out]
      n193 = call-poly <vilib>:"WPI_RobotDriveArcadeDrive.vi"("Y axis value"=0.25 ("X axis value"), "X axis value"=0.5, "RobotDriveDevRef"=w306) -> ("Motor Values"=w298:dbl[], "RobotDriveDevRef"=w305:T15)  [unwired: 1 in, 6 out]
      n194 = call <vilib>:"SD Write Numeric Array.vi"("Numeric Array"=w298, "Name"=w296) -> ()  [unwired: 8 in, 2 out]
      n195 = call <vilib>:"WPI_RobotDriveDelayAndUpdateSafety.vi"("Delay (s)"=0.5, "RobotDriveDevRef"=w305) -> ("RobotDriveDevRef 2"=w304:T15)  [unwired: 8 in, 1 out]
      n196 = call-poly <vilib>:"WPI_RobotDriveArcadeDrive.vi"("Y axis value"=0.0 ("X axis value"), "X axis value"=0.0, "RobotDriveDevRef"=w304) -> ("Motor Values"=w297:dbl[])  [unwired: 1 in, 7 out]
      n197 = call <vilib>:"SD Write Numeric Array.vi"("Numeric Array"=w297, "Name"=w296) -> ()  [unwired: 8 in, 2 out]
    }
    frame Enabled {
    }
  }
  n198 = disable-structure shown="Disabled" {
    frame Disabled {
      # "This sample code describes robot movements in an array. You can extend it to control other motors\non your robot. You can also use file I/O to move the data to a text file."
      n199 = call <vilib>:"WPI_RobotDriveRefNum Registry Get.vi"("refnum name"="Left and Right Motors") -> ("RobotDriveDevRef"=w315:T15)  [unwired: 1 in, 9 out]
      n200 = for {
        shift-right: [w321] -> _
        shift-left: w315 -> [w322]
        tunnel: "Array of robot movements" -> [w317] mode=indexing
        n201 = Unbundle By Name(w317) -> ("X Joystick Value"=w320:dbl, "Y Joystick Value"=w319:dbl, "Delay (sec)"=w318:dbl)  [unwired: 1 out]
        n202 = call-poly <vilib>:"WPI_RobotDriveArcadeDrive.vi"("Y axis value"=w319, "X axis value"=w320, "RobotDriveDevRef"=w322) -> ("Motor Values"=w324:dbl[], "RobotDriveDevRef"=w323:T15)  [unwired: 1 in, 6 out]
        n203 = call <vilib>:"SD Write Numeric Array.vi"("Numeric Array"=w324, "Name"="RobotDrive Motors") -> ()  [unwired: 8 in, 2 out]
        n204 = call <vilib>:"WPI_RobotDriveDelayAndUpdateSafety.vi"("Delay (s)"=w318, "RobotDriveDevRef"=w323) -> ("RobotDriveDevRef 2"=w321:T15)  [unwired: 8 in, 1 out]
        "Current Movement, for debugging" <- w317
      }
    }
    frame Enabled {
    }
  }
